vi "Dashboard Main.vi"() -> ()   [LabVIEW 2011]
uses:
  Shared/Shifter State.ctl
  Shared/Shooter Control Mode.ctl
  Shared/Dashboard Datatype.ctl
  Shared/Drive Base Dashboard Package.ctl
  Shared/Shooter Dashboard Package.ctl
  Shared/cRIO Performance Details.ctl
  Dashboard Global Data.vi
panel:
  in  "Show\nSpeed & RPM":bool
  out "Shooter RPM Small":dbl(knob) scale=0.0..6000.0 scale format="%#_6p"
  out "Motor Speed Small":dbl(knob) scale=0.0..100.0 scale format="%#_6p%%"
  out "Motor Speed":dbl(knob) caption="Set Speed" scale=0.0..100.0 scale format="%#_6p%%"
  out "Shooter RPM":dbl(knob) caption="Current RPM" scale=0.0..6000.0 scale format="%#_6p"
  out "Shooter Cluster":cluster{dbl, dbl}(knob) caption="Set RPM" scale=0.0..6000.0 scale format="%#_6p"
  out "Shooter Mode":T1=enum."Off"
  out "CPU":u8(slide) scale=0.0..100.0
  out "Flash":u8(slide) scale=0.0..100.0
  out "RAM":u8(slide) scale=0.0..100.0
  out "Gear Box":T2
  out "Left":dbl(slide) scale=-1.0..1.0
  out "Right":dbl(slide) scale=-1.0..1.0
  out "Camera Image":T3(plugin-control)
  out "Dashboard Datatype Warning":string="Warning: The Dashboard Datatype used by the robot project and this dashboard do not match.\nSee diagram for more details."
  out "Image Error Message":string="Timeout in Camera Communications"
  # "Aiminright"
  # "2012"
  # "Shooter RPM"
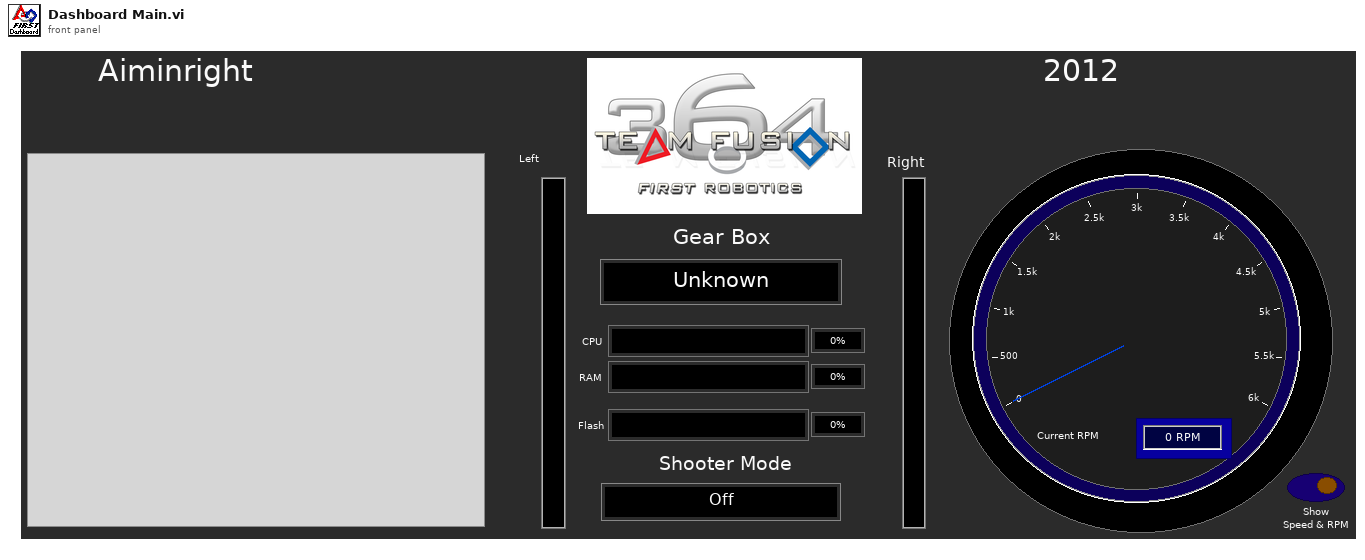
[diagram p1: front panel]
types:
  T1 = typedef "Shooter Control Mode.ctl" = enum16{"Key", "Mid Field", "Backfield", "Topspin", "Open Loop Control", "Off"}
  T2 = typedef "Shifter State.ctl" = enum16{"Unknown", "Low", "High"}
  T3 = typedef "IMAQ Image.ctl" = refnum<image>
  T4 = typedef "Dashboard Datatype.ctl" = cluster{"Drive Base":T5, "Shooter":T6, "Performance Details":T7}
  T5 = typedef "Drive Base Dashboard Package.ctl" = cluster{"Left":dbl, "Right":dbl, "Shifter":T2}
  T6 = typedef "Shooter Dashboard Package.ctl" = cluster{"Set RPM":dbl, "Current RPM":dbl, "Motor Speed":dbl, "Shooter Mode":enum16{"Off", "Open Loop Control", "Closed Loop Control", "Top Spin"}, "Shooter Speed Enumerated Type":T1}
  T7 = typedef "cRIO Performance Details.ctl" = cluster{"CPU Utilization":dbl, "RAM total (bytes)":u32, "RAM available (bytes)":u32, "Flash size (bytes)":i64, "Flash free (bytes)":i64}
  T8 = typedef "Image Type" = u32
  T9 = typedef "LVRectTypeDef.ctl" = cluster{"left":i16, "top":i16, "right":i16, "bottom":i16}
  T10 = enum16{"Off", "Open Loop Control", "Closed Loop Control", "Top Spin"}
  T11 = cluster{"Competition mode":bool, "Robot Link":bool, "Autonomous":bool, "Enabled":bool, "E-Stop":bool}
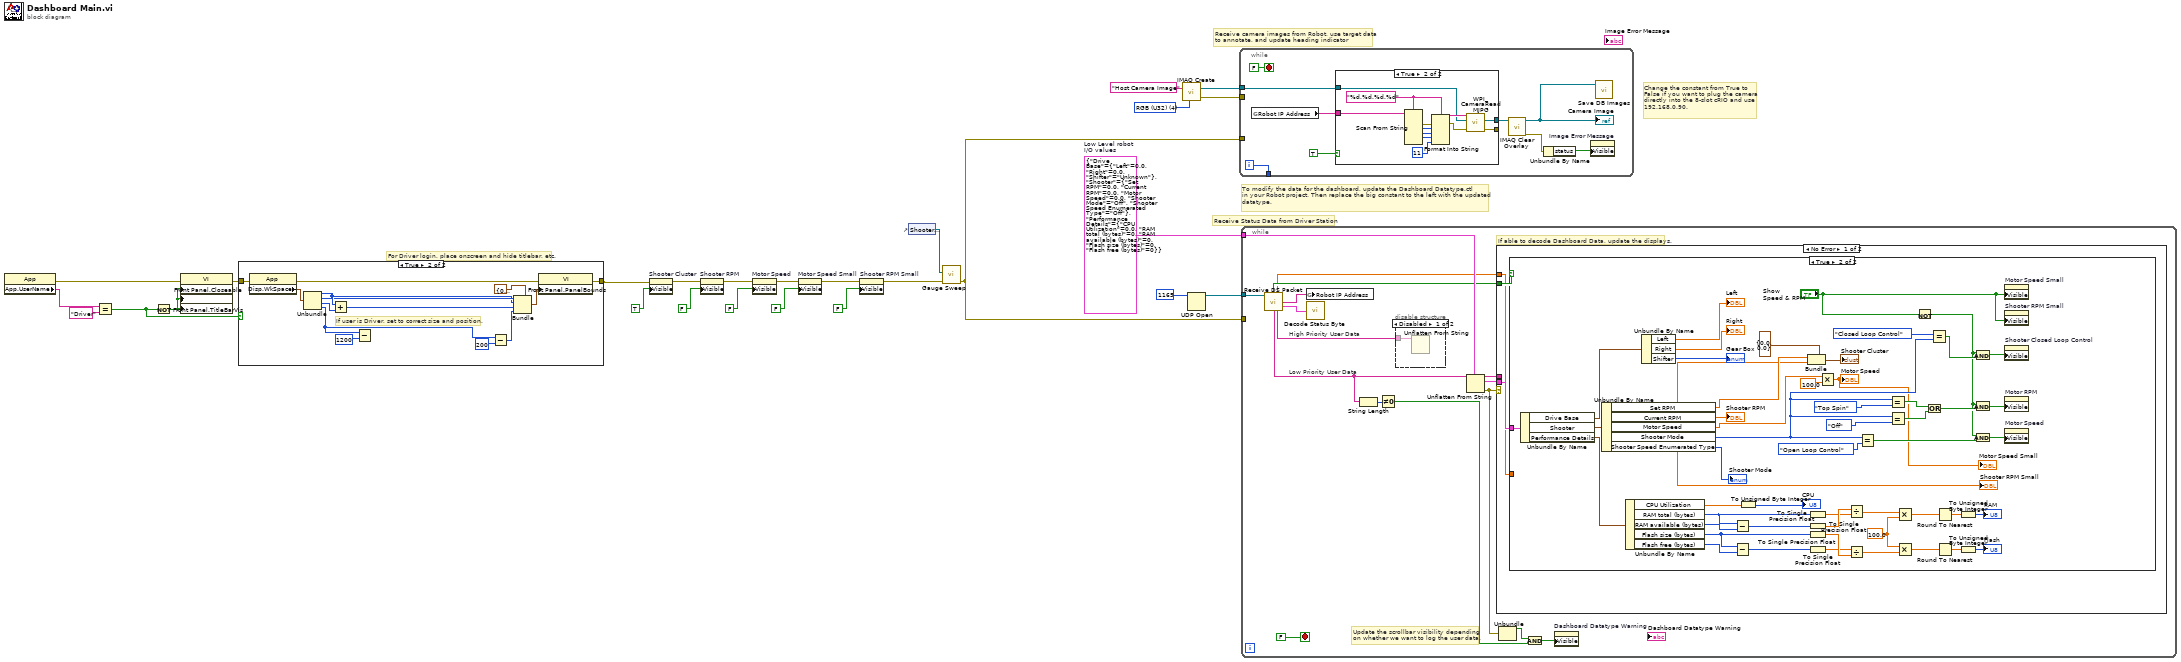
[diagram p0: block diagram]
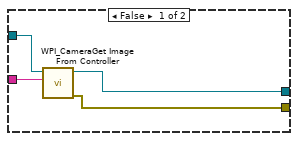
[diagram p5: hidden frame]
diagram:
  w16 = T4 {"Drive Base"={"Left"=0.0, "Right"=0.0, "Shifter"=enum."Unknown"}, "Shooter"={"Set RPM"=0.0, "Current RPM"=0.0, "Motor Speed"=0.0, "Shooter Mode"=enum."Off", "Shooter Speed Enumerated Type"=enum."Off"}, "Performance Details"={"CPU Utilization"=0.0, "RAM total (bytes)"=0, "RAM available (bytes)"=0, "Flash size (bytes)"=0, "Flash free (bytes)"=0}}  # Low Level robot I/O values
  w20 = T8 4 items=["Grayscale (U8)", "Grayscale (I16)", "Grayscale (SGL)", "Complex (CSG)", "RGB (U32)", "HSL (U32)", "RGB (U64)"] ("Image Type")
  # "Change the constant from True to\nFalse if you want to plug the camera\ndirectly into the 8-slot cRIO and use\n192.168.0.90."
  # "To modify the data for the dashboard, update the Dashboard Datatype.ctl\nin your Robot project. Then replace the big constant to the left with the updated\ndatatype."
  # "Receive Status Data from Driver Station"
  # "Receive camera images from Robot, use target data\nto annotate, and update heading indicator"
  # "For Driver login, place onscreen and hide titlebar, etc."
  n1 = property class="App"() -> (error out=w7:errorcluster, "App.UserName"=w24:string)  [unwired: 2 in, 1 out]
  n2 = Equal?(x=w24, y="Driver") -> (x = y?=w25:bool)
  n3 = Not(x=w25) -> (.not. x?=w26:bool)
  n4 = property class="VI"(error in=w7, "Front Panel.Closeable"=w26, "Front Panel.Minimizeable"=w26, "Front Panel.TitleBarVis"=w26) -> (error out=w15:errorcluster)  [unwired: 1 in, 1 out]
  n5 = case shown="True" w25 {
    tunnel: [w27 w30] -> w3
    tunnel: w15 -> [w27 w28]
    frame False {
    }
    frame True {
      # "If user is Driver, set to correct size and position."
      n6 = property class="App"(error in=w28) -> (error out=w29:errorcluster, "Disp.WkSpace"=w41:T9)  [unwired: 1 in, 1 out]
      n7 = Unbundle(w41) -> ("left"=w37:i16, "top"=w31:i16, "right"=w32:i16, "bottom"=w34:i16)
      n8 = Add(x=w37, y=w32) -> (x+y=w38:i16)
      n9 = Subtract(x=w34, y=1200) -> ()  [unwired: 1 out]
      n10 = Subtract(x=w34, y=200) -> (x-y=w35:i32)
      n11 = Bundle(cluster=cluster{"left":i16, i32, i32, i32} {"left"=0, 0, 0, 0} ("output cluster"), "left"=w37, w31, w38, w35) -> (w40:cluster{"left":i16, i32, i32, i32})
      n12 = property class="VI"(error in=w29, "Front Panel.PanelBounds"=w40) -> (error out=w30:errorcluster)  [unwired: 1 in, 1 out]
    }
  }
  n13 = property on="Shooter Cluster" class="Knob (strict)"(error in=w3, "Visible"=TRUE) -> (error out=w9:errorcluster)  [unwired: 1 in, 1 out]
  n14 = property on="Shooter RPM" class="Knob (strict)"(error in=w9, "Visible"=FALSE) -> (error out=w8:errorcluster)  [unwired: 1 in, 1 out]
  n15 = property on="Motor Speed" class="Knob (strict)"(error in=w8, "Visible"=FALSE) -> (error out=w6:errorcluster)  [unwired: 1 in, 1 out]
  n16 = property on="Motor Speed Small" class="Knob (strict)"(error in=w6, "Visible"=FALSE) -> (error out=w5:errorcluster)  [unwired: 1 in, 1 out]
  n17 = property on="Shooter RPM Small" class="Knob (strict)"(error in=w5, "Visible"=FALSE) -> (error out=w4:errorcluster)  [unwired: 1 in, 1 out]
  n18 = control-ref of="Shooter Cluster"() -> (w13:refnum<vi>)
  n19 = call "Gauge Sweep.vi"("error in (no error)"=w4, "Ctl Refnum"=w13) -> ("error out"=w14:errorcluster)  [unwired: 9 in]
  n20 = call "IMAQ Create"("Image Name"="Host Camera Image", "Image Type"=w20) -> ("New Image"=w18:T3, "error out"=w17:errorcluster)  [unwired: 2 in, 1 out]
  n21 = UDP Open(11:u16 1165 ("port")) -> (port=w21:refnum<k16>)  [unwired: 2 in, 4 out]
  n22 = while {
    tunnel: w18 -> [w49]
    tunnel: w17 -> [_]
    tunnel: [w47] -> _
    tunnel: w14 -> [_]
    i -> [w47]
    stop <- FALSE stop-if-true
    n23 = global read "Dashboard Global Data.vi" "Robot IP Address"() -> (w42:string)
    n24 = case shown="True" TRUE {
      tunnel: w49 -> [w53 w60]
      tunnel: [w51 w58] -> _
      tunnel: [w52 w59] -> w44
      tunnel: w42 -> [w54 w63]
      frame False {
        n25 = call <vilib>:"WPI_CameraGet Image From Controller.vi"("Controller Address"=w54, "Image"=w53) -> ("error out"=w51:errorcluster, "Image Out"=w52:T3)  [unwired: 2 in, 6 out]
      }
      frame True {
        w55 = "%d.%d.%d.%d" ("format string")
        n26 = Scan From String(format string=w55, input string=w63) -> (error out=w62:errorcluster, output 1=w64:i32, output 2=w65:i32, output 3=w66:i32)  [unwired: 2 in, 7 out]
        n27 = Format Into String(format string=w55, error in=w62, w64, w65, w66, 11 ("IP Suffix:")) -> (resulting string=w61:string, error out=w57:errorcluster)  [unwired: 1 in]
        n28 = call <vilib>:"WPI_CameraRead MJPG.vi"("error in"=w57, "Image"=w60, "address"=w61) -> ("error out"=w58:errorcluster, "Image Out"=w59:T3)  [unwired: 7 in]
      }
    }
    n29 = call "IMAQ Clear Overlay"("Image"=w44) -> ("error out"=w45:errorcluster, "Image Out"=w43:T3)  [unwired: 2 in, 7 out]
    "Camera Image" <- w43
    n30 = Unbundle By Name(w45) -> ("status"=w46:bool)
    n31 = property on="Image Error Message" class="Str"("Visible"=w46) -> ()  [unwired: 2 in, 2 out]
    n32 = call "Save DB Images.vi"("Image"=w43) -> ()  [unwired: 2 in, 1 out]
  }
  n33 = while {
    tunnel: w21 -> [w80]
    tunnel: w16 -> [w79]
    tunnel: w14 -> [_]
    stop <- FALSE stop-if-true
    # "High Priority User Data"
    # "Low Priority User Data"
    # "Update the scrollbar visibility depending\non whether we want to log the user data."
    # "If able to decode Dashboard Data, update the displays."
    n34 = call "Receive DS Packet.vi"("Recv Socket"=w80) -> ("New Dashboard Data"=w76:bool, "Battery"=w68:sgl, "Robot IP Address"=w67:string, "Status"=w81:T11, "Low Priority User Data"=w70:string, "High Priority User Data"=w69:string)  [unwired: 1 in, 8 out]
    n35 = global write "Dashboard Global Data.vi" "Robot IP Address"(w67) -> ()
    n36 = call "Decode Status Byte.vi"("Status Byte"=w81) -> ()  [unwired: 2 out]
    n37 = String Length(string=w70) -> (length=w71:i32)
    n38 = Not Equal To 0?(x=w71) -> (x != 0?=w74:bool)
    n39 = disable-structure shown="Disabled" {
      disable-tunnel: w69 -> [w83 _]
      frame Disabled {
        n40 = Unflatten From String(binary string=w83) -> ()  [unwired: 2 in, 5 out]
      }
      frame Enabled {
      }
    }
    n41 = Unflatten From String(type=w79, binary string=w70) -> (rest of the binary string=w72:string, value=w78:T4, error out=w77:errorcluster)  [unwired: 1 in, 2 out]
    n42 = case shown="No Error" w77 {
      tunnel: w78 -> [w86 _]
      tunnel: w76 -> [w85 _]
      tunnel: w72 -> [_ _]
      tunnel: w68 -> [w84 _]
      frame No Error {
        n43 = case shown="True" w85 {
          tunnel: w86 -> [_ w134]
          tunnel: w84 -> [_ _]
          frame False {
            # "Don't update if the robot hasn't sent new data"
          }
          frame True {
            w122 = sgl 100.0
            n44 = Unbundle By Name(w134) -> ("Drive Base"=w136:T5, "Shooter"=w137:T6, "Performance Details"=w135:T7)
            n45 = Unbundle By Name(w137) -> ("Set RPM"=w107:dbl, "Current RPM"=w87:dbl, "Motor Speed"=w106:dbl, "Shooter Mode"=w99:T10, "Shooter Speed Enumerated Type"=→"Shooter Mode":T1)
            "Shooter RPM" <- w87
            "Shooter RPM Small" <- w87
            n46 = Unbundle By Name(w135) -> ("CPU Utilization"=w114:dbl, "RAM total (bytes)"=w128:u32, "RAM available (bytes)"=w131:u32, "Flash size (bytes)"=w113:i64, "Flash free (bytes)"=w130:i64)
            n47 = Unbundle By Name(w136) -> ("Left"=→"Left":dbl, "Right"=→"Right":dbl, "Shifter"=→"Gear Box":T2)
            n48 = Subtract(x=w128, y=w131) -> (x-y=w129:u32)
            n49 = Subtract(x=w113, y=w130) -> (x-y=w127:i64)
            n50 = To Unsigned Byte Integer(number=w114) -> (unsigned 8bit integer=→"CPU":u8)
            n51 = Bundle(cluster=cluster{dbl, dbl} {0.0, 0.0} ("Shooter RPM"), w107, w87) -> (→"Shooter Cluster":cluster{dbl, dbl})
            n52 = To Single Precision Float(number=w128) -> (single precision float=w125:sgl)
            n53 = To Single Precision Float(number=w129) -> (single precision float=w126:sgl)
            n54 = To Single Precision Float(number=w113) -> (single precision float=w112:sgl)
            n55 = To Single Precision Float(number=w127) -> (single precision float=w111:sgl)
            n56 = Multiply(x=w106, y=100.0) -> (x*y=→"Motor Speed" →"Motor Speed Small":dbl)
            n57 = Divide(x=w126, y=w125) -> (x/y=w124:sgl)
            n58 = Divide(x=w111, y=w112) -> (x/y=w123:sgl)
            n59 = Equal?(x=w99, y=T10."Open Loop Control") -> (x = y?=w97:bool)
            n60 = Equal?(x=w99, y=T10."Top Spin") -> (x = y?=w101:bool)
            n61 = Equal?(x=w99, y=T10."Off") -> (x = y?=w96:bool)
            n62 = Multiply(x=w124, y=w122) -> (x*y=w121:sgl)
            n63 = Multiply(x=w122, y=w123) -> (x*y=w120:sgl)
            n64 = Not(x="Show\nSpeed & RPM") -> (.not. x?=w90:bool)
            n65 = Or(x=w101, y=w96) -> (x .or. y?=w92:bool)
            n66 = Equal?(x=T10."Closed Loop Control" ("Shooter Mode"), y=w99) -> (x = y?=w105:bool)
            n67 = Round To Nearest(number=w121) -> (nearest integer value=w119:sgl)
            n68 = Round To Nearest(number=w120) -> (nearest integer value=w118:sgl)
            n69 = To Unsigned Byte Integer(number=w119) -> (unsigned 8bit integer=→"RAM":u8)
            n70 = To Unsigned Byte Integer(number=w118) -> (unsigned 8bit integer=→"Flash":u8)
            n71 = And(x=w90, y=w105) -> (x .and. y?=w94:bool)
            n72 = And(x=w90, y=w92) -> (x .and. y?=w93:bool)
            n73 = And(x=w90, y=w97) -> (x .and. y?=w91:bool)
            n74 = property on="Motor Speed Small" class="Knob (strict)"("Visible"="Show\nSpeed & RPM") -> ()  [unwired: 2 in, 2 out]
            n75 = property on="Shooter RPM Small" class="Knob (strict)"("Visible"="Show\nSpeed & RPM") -> ()  [unwired: 2 in, 2 out]
            n76 = property on="Shooter Closed Loop Control" class="Knob (strict)"("Visible"=w94) -> ()  [unwired: 2 in, 2 out]
            n77 = property on="Motor RPM" class="Knob (strict)"("Visible"=w93) -> ()  [unwired: 2 in, 2 out]
            n78 = property on="Motor Speed" class="Knob (strict)"("Visible"=w91) -> ()  [unwired: 2 in, 2 out]
          }
        }
      }
      frame Error {
        # "Your datatypes don't match. The Dashboard Datatype.ctl in your Robot project\nand the big constant to the left of the loop need to match."
      }
    }
    n79 = Unbundle(w77) -> ("status"=w73:bool)  [unwired: 2 out]
    n80 = And(x=w73, y=w74) -> (x .and. y?=w75:bool)
    n81 = property on="Dashboard Datatype Warning" class="Str"("Visible"=w75) -> ()  [unwired: 2 in, 2 out]
  }
